vi "PhaseSpace_wrist.vi"() -> ()   [LabVIEW 2014]
uses:
  lib/libowlsock.dll
panel:
  out "output array":sgl[](array[numeric])=[0.3378775, -0.412445, 0.36083448, 0.0, 0.0, 0.0, 0.0, 0.0, 0.0]
  out "String":string="0.338,-0.412,0.361,0.000,0.000,0.000,0.000,0.000,0.000,"
  out "frame":i32=1194
  in  "Occulus address":string="localhost"
  in  "OC2":u8=1
  in  "OC3":u8=2
  in  "OC1":u8
  in  "Stop":bool=TRUE
  out "data":sgl[][](array[numeric])=[[272.08093, 8.818391, 616.6266], [358.27786, -2.124915, 632.85004], [332.61215, -2.6014774, 569.41797], [472.55515, -720.1108, 521.30414], [483.88748, -615.3709, 459.3937], [398.05954, -371.48962, 482.48965], [0.0, 0.0, 0.0], [469.56293, -662.9195, 501.45453], [0.0, 0.0, 0.0], [0.0, 0.0, 0.0], [0.0, 0.0, 0.0], [0.0, 0.0, 0.0], [0.0, 0.0, 0.0], [0.0, 0.0, 0.0], [0.0, 0.0, 0.0], [0.0, 0.0, 0.0], [0.0, 0.0, 0.0], [0.0, 0.0, 0.0], [0.0, 0.0, 0.0], [0.0, 0.0, 0.0], [0.0, 0.0, 0.0], [0.0, 0.0, 0.0], [0.0, 0.0, 0.0], [0.0, 0.0, 0.0], [0.0, 0.0, 0.0], [0.0, 0.0, 0.0], [0.0, 0.0, 0.0], [0.0, 0.0, 0.0], [0.0, 0.0, 0.0], [0.0, 0.0, 0.0], [0.0, 0.0, 0.0], [0.0, 0.0, 0.0]]
  out "connected\nto server?":bool=TRUE
  in  "server address":string="192.168.0.101"
  # "wrist"
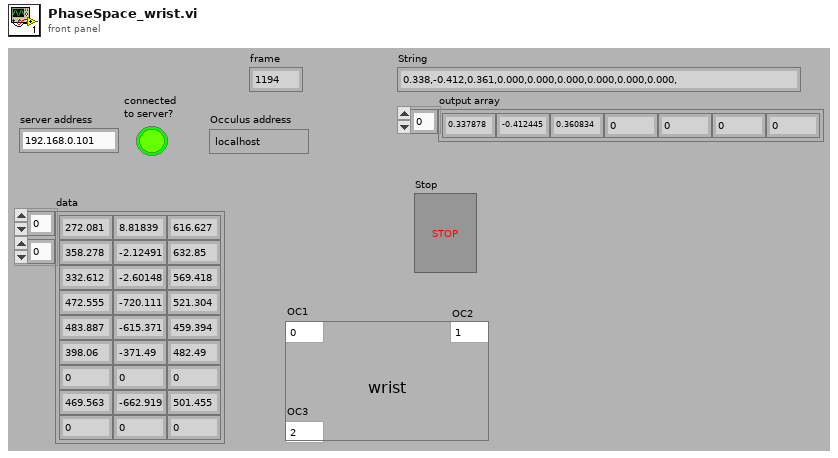
[diagram p1: front panel]
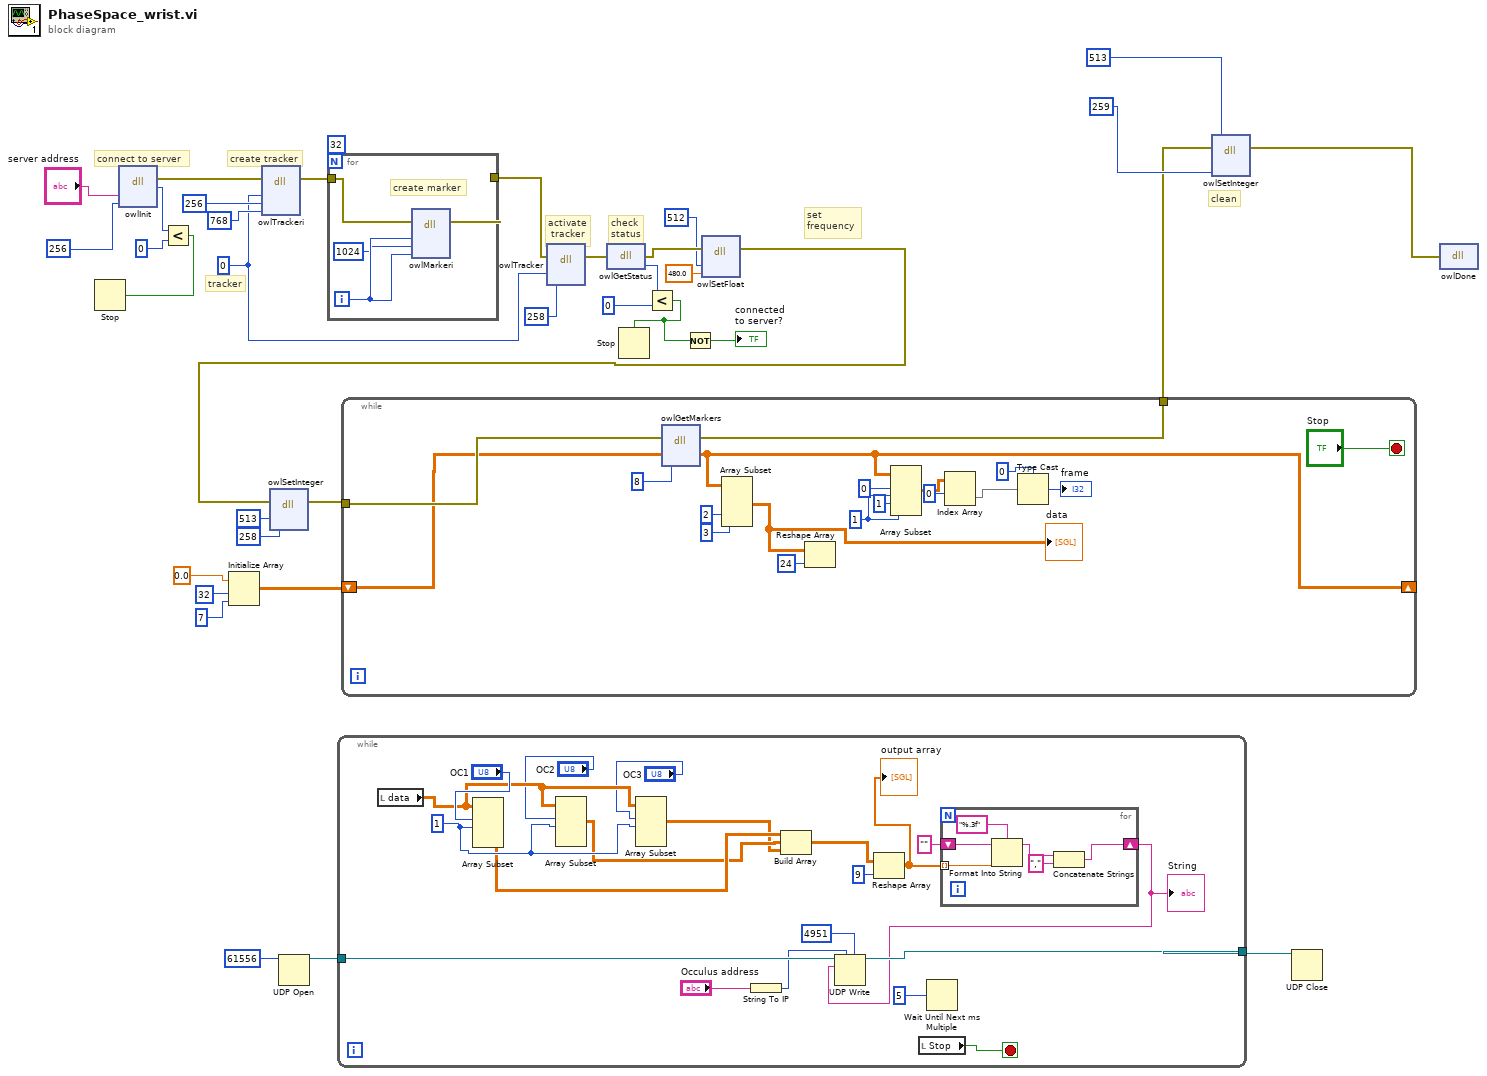
[diagram p0: block diagram]
diagram:
  w28 = i16 0 ("y")
  # "set\nfrequency"
  # "check\nstatus"
  # "activate\n tracker"
  # "tracker"
  # "clean"
  # "create tracker"
  # "connect to server"
  n1 = dll-call lib="C:/Users/qiushifu/Desktop/MyoPythonProgram/PSClientSDK/lib/libowlsock.dll" fn="owlInit"("server"="server address", "flags"=i16 256) -> (error out=w33:errorcluster, "return type"=w34:i16)  [unwired: 4 in, 2 out]
  n2 = Less?(x=w34, y=i16 0) -> (x < y?=w22:bool)
  n3 = Stop(stop? (T)=w22) -> ()
  n4 = Initialize Array(sgl 0.0, 32, 7) -> (w12:sgl[][])
  n5 = dll-call lib="C:/Users/qiushifu/Desktop/MyoPythonProgram/PSClientSDK/lib/libowlsock.dll" fn="owlTrackeri"(error in=w33, "tracker"=w28, "pname"=i16 256 ("flags"), "param"=i16 768 ("flags")) -> (error out=w30:errorcluster)  [unwired: 5 in, 2 out]
  n6 = UDP Open(11:u16 61556 ("port")) -> (port=w3:refnum<k16>)  [unwired: 1 in, 5 out]
  n7 = for {
    N: 32 -> [_]
    tunnel: w30 -> [w38]
    tunnel: [w37] -> w27
    i -> [w40]
    # "create marker"
    n8 = dll-call lib="C:/Users/qiushifu/Desktop/MyoPythonProgram/PSClientSDK/lib/libowlsock.dll" fn="owlMarkeri"(error in=w38, "marker"=w40, "pname"=i16 1024 ("flags"), "param"=w40) -> (error out=w37:errorcluster)  [unwired: 3 in, 4 out]
  }
  n9 = while {
    tunnel: w3 -> [w55]
    tunnel: [w54] -> w2
    stop <- w46 stop-if-true
    w58 = 1 ("length")
    n10 = local read "data"() -> (w59:sgl[][])
    n11 = Array Subset(array=w59, index (row)="OC1", length (row)=w58) -> (w45:sgl[][])  [unwired: 2 in]
    n12 = Array Subset(array=w59, index (row)="OC2", length (row)=w58) -> (w44:sgl[][])  [unwired: 2 in]
    n13 = Array Subset(array=w59, index (row)="OC3", length (row)=w58) -> (w43:sgl[][])  [unwired: 2 in]
    n14 = String To IP(1:"Occulus address") -> (0:w51:u32)
    n15 = Build Array(w45, w44, w43) -> (w42:sgl[][][])
    n16 = Reshape Array(w42, 9 ("dimension size")) -> (w41:sgl[])
    "output array" <- w41
    n17 = local read "Stop"() -> (w46:bool)
    n18 = Wait Until Next ms Multiple(millisecond multiple=u32 5 ("milliseconds to wait")) -> ()  [unwired: 1 out]
    n19 = for {
      shift-right: [w63] -> w47
      shift-left: "" -> [w65]
      tunnel: w41 -> [w61] mode=indexing
      n20 = Format Into String(format string="%.3f", initial string=w65, w61) -> (resulting string=w64:string)  [unwired: 1 in, 1 out]
      n21 = Concatenate Strings(w64, "," ("string")) -> (w63:string)
    }
    "String" <- w47
    n22 = UDP Write(address=w51, port or service name=u16 4951 ("port"), connection ID=w55, data in=w47) -> (3:w54:refnum<k16>)  [unwired: 1 in, 2 out]
  }
  n23 = dll-call lib="C:/Users/qiushifu/Desktop/MyoPythonProgram/PSClientSDK/lib/libowlsock.dll" fn="owlTracker"(error in=w27, "tracker"=w28, "pname"=i16 258 ("flags")) -> (error out=w25:errorcluster)  [unwired: 4 in, 2 out]
  n24 = dll-call lib="C:/Users/qiushifu/Desktop/MyoPythonProgram/PSClientSDK/lib/libowlsock.dll" fn="owlGetStatus"(error in=w25) -> (error out=w21:errorcluster, "return type"=w23:u16)  [unwired: 2 in, 1 out]
  n25 = Less?(x=w23, y=i16 0) -> (x < y?=w17:bool)
  n26 = Stop(stop? (T)=w17) -> ()
  n27 = Not(x=w17) -> (.not. x?=→"connected\nto server?":bool)
  n28 = dll-call lib="C:/Users/qiushifu/Desktop/MyoPythonProgram/PSClientSDK/lib/libowlsock.dll" fn="owlSetFloat"(error in=w21, "pname"=u16 512, "param"=sgl 480.0) -> (error out=w9:errorcluster)  [unwired: 4 in, 2 out]
  n29 = dll-call lib="C:/Users/qiushifu/Desktop/MyoPythonProgram/PSClientSDK/lib/libowlsock.dll" fn="owlSetInteger"(error in=w9, "pname"=u16 513, "param"=u16 258) -> (error out=w8:errorcluster)  [unwired: 4 in, 2 out]
  n30 = while {
    tunnel: w8 -> [w83]
    tunnel: [w80] -> w4
    shift-right: [w76] -> _
    shift-left: w12 -> [w82]
    stop <- "Stop" stop-if-true
    w74 = 1 ("length")
    n31 = dll-call lib="C:/Users/qiushifu/Desktop/MyoPythonProgram/PSClientSDK/lib/libowlsock.dll" fn="owlGetMarkers"(error in=w83, "markers"=w82, "count"=u16 8) -> (error out=w80:errorcluster, "markers"=w76:sgl[][])  [unwired: 3 in, 2 out]
    n32 = Array Subset(array=w76, index (col)=2 ("index"), length (col)=3 ("length")) -> (w67:sgl[][])  [unwired: 2 in]
    "data" <- w67
    n33 = Reshape Array(w67, 24 ("dimension size")) -> ()  [unwired: 1 out]
    n34 = Array Subset(array=w76, index (row)=0 ("length"), length (row)=w74, index (col)=1 ("index"), length (col)=w74) -> (w72:sgl[][])
    n35 = Index Array(array=w72, index (row)=0) -> (element=w70:sgl[])  [unwired: 1 in]
    n36 = Type Cast(type=0 ("index (row)"), x=w70) -> (*(type *) &x=→"frame":i32)
  }
  n37 = dll-call lib="C:/Users/qiushifu/Desktop/MyoPythonProgram/PSClientSDK/lib/libowlsock.dll" fn="owlSetInteger"(error in=w4, "pname"=u16 513, "param"=u16 259 ("pname")) -> (error out=w5:errorcluster)  [unwired: 4 in, 2 out]
  n38 = UDP Close(connection ID=w2) -> ()  [unwired: 1 in, 2 out]
  n39 = dll-call lib="C:/Users/qiushifu/Desktop/MyoPythonProgram/PSClientSDK/lib/libowlsock.dll" fn="owlDone"(error in=w5) -> ()  [unwired: 2 in, 3 out]
